vi "Przebiegi_edycja_math.vi"(8 "error in (no error)":errorcluster, 11 "Wektor przebiegow in":waveform(dbl)[](array[waveform])) -> (0 "error out":errorcluster, 3 "Wektor przebiegow out":waveform(dbl)[](array[waveform]))   [LabVIEW 2013]
doc: "Realizuje funkcję\nf(x) = a * sygnał + b\nna wybranym przebiegu"
panel:
  in  "C":dbl
  in  "Przebieg C":i32(ring) items=["Przebieg 0", "Przebieg 1", "Przebieg 2", "Przebieg 3", "Stała"]
  in  "Przebieg B":i32(ring) items=["Przebieg 0", "Przebieg 1", "Przebieg 2", "Przebieg 3", "Stała"]
  out "Funkcja":string
  in  "B":dbl=1.0
  in  "A":dbl=1.0
  in  "OK Button":bool
  in  "Cancel Button":bool
  in  "Przebieg A":i32(ring) items=["Przebieg 0", "Przebieg 1", "Przebieg 2", "Przebieg 3", "Stała"]
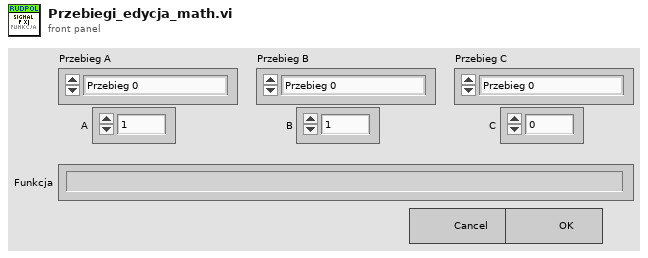
[diagram p1: front panel]
types:
  T1 = cluster{"Przebieg A":i32, "Przebieg B":i32, "Przebieg C":i32, "A":dbl, "B":dbl, "C":dbl}
  T2 = typedef "LVStringsAndValuesArrayTypeDef_I32.ctl" = cluster{"String":string, "Value":i32}[]
  T3 = cluster{"StringsAndValues[]":T2, "StringsAndValues[]":T2, "StringsAndValues[]":T2}
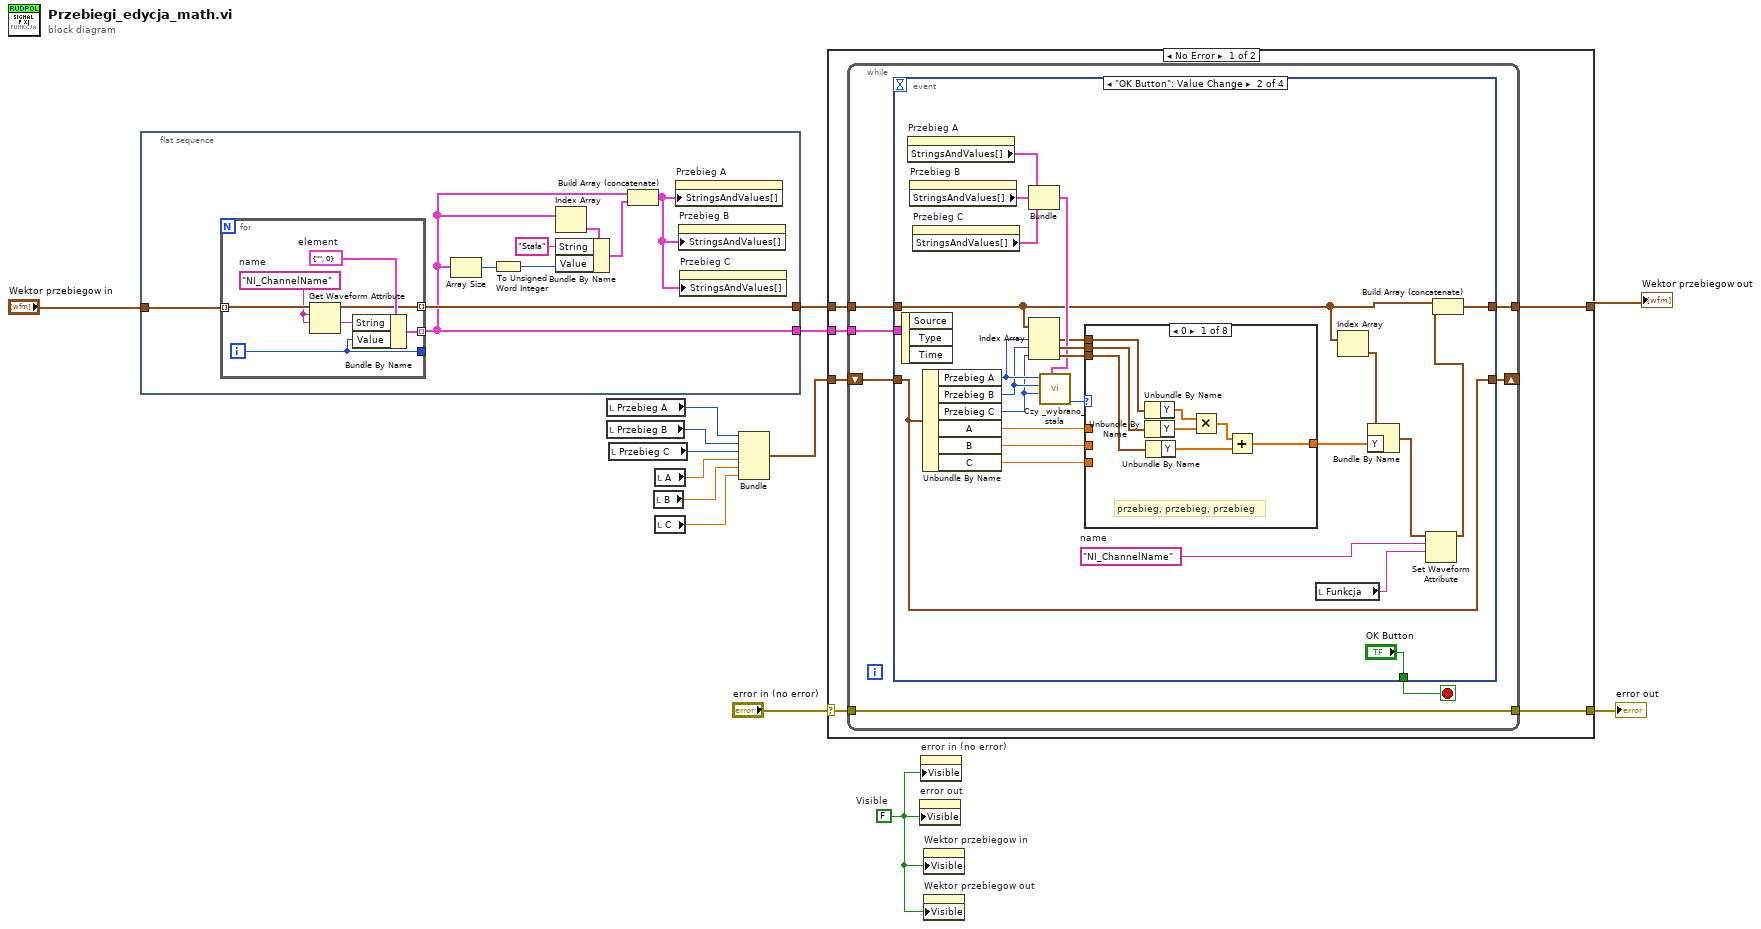
[diagram p0: block diagram]
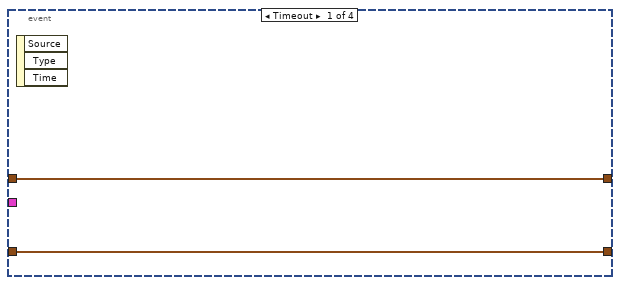
[diagram p2: hidden frame]
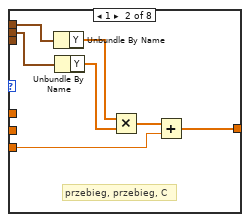
[diagram p3: hidden frame]
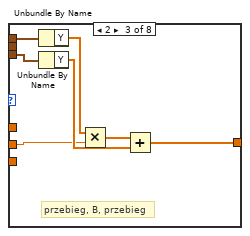
[diagram p4: hidden frame]
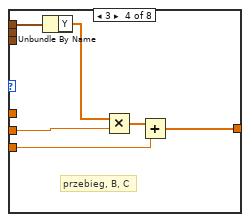
[diagram p5: hidden frame]
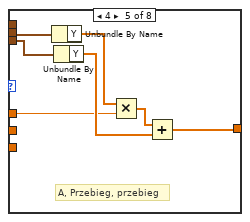
[diagram p6: hidden frame]
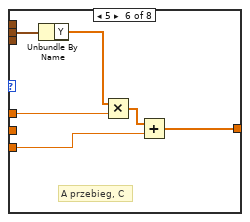
[diagram p7: hidden frame]
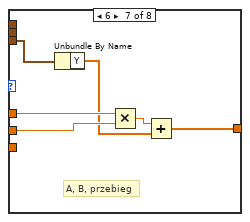
[diagram p8: hidden frame]
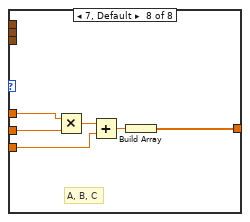
[diagram p9: hidden frame]
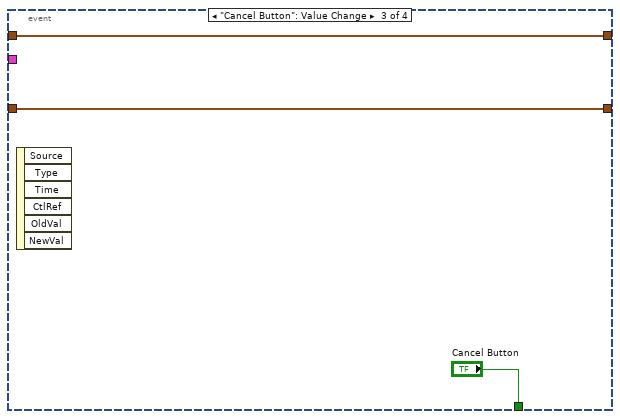
[diagram p10: hidden frame]
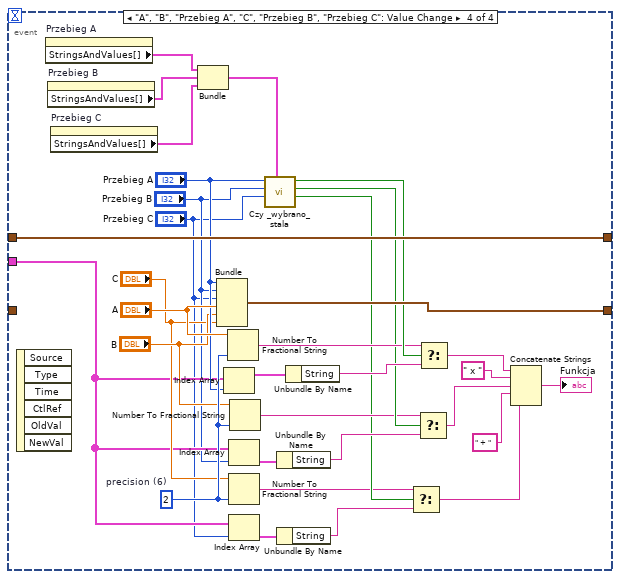
[diagram p11: hidden frame]
diagram:
  w8 = FALSE  # Visible
  n1 = flat-sequence {
    tunnel: "Wektor przebiegow in" -> [w23]
    tunnel: [w18] -> w11
    tunnel: [w22] -> w10
    frame #0 {
      n2 = for {
        tunnel: w23 -> [w30] mode=indexing
        tunnel: [w26] -> _
        tunnel: [w25] -> w18 mode=indexing
        tunnel: [w24] -> w22 mode=indexing
        i -> [w26]
        w28 = cluster{"String":string, "Value":u16} {"String"="", "Value"=0}  # element
        w29 = "NI_ChannelName"  # name
        n3 = Get Waveform Attribute(5:w29, 6:w29, 7:w30) -> (1:w27:string, 3:w24:waveform(dbl))  [unwired: 1 in, 2 out]
        n4 = Bundle By Name(cluster=w28, "String"=w27, "Value"=w26) -> (w25:cluster{"String":string, "Value":u16})
      }
      n5 = Array Size(array=w18) -> (size(s)=w17:i32)
      n6 = To Unsigned Word Integer(number=w17) -> (unsigned 16bit integer=w16:u16)
      n7 = Index Array(array=w18) -> (element=w21:cluster{"String":string, "Value":u16})  [unwired: 1 in]
      n8 = Bundle By Name(cluster=w21, "String"="Stała", "Value"=w16) -> (w20:cluster{"String":string, "Value":u16})
      n9 = Build Array (concatenate)(w18, w20) -> (w15:cluster{"String":string, "Value":u16}[])
      n10 = property on="Przebieg A" class="Ring (strict)"("StringsAndValues[]"=w15) -> ()  [unwired: 2 in, 2 out]
      n11 = property on="Przebieg B" class="Ring (strict)"("StringsAndValues[]"=w15) -> ()  [unwired: 2 in, 2 out]
      n12 = property on="Przebieg C" class="Ring (strict)"("StringsAndValues[]"=w15) -> ()  [unwired: 2 in, 2 out]
    }
  }
  n13 = local read "Przebieg A"() -> (w7:i32)
  n14 = local read "Przebieg B"() -> (w2:i32)
  n15 = local read "Przebieg C"() -> (w1:i32)
  n16 = local read "B"() -> (w4:dbl)
  n17 = local read "A"() -> (w5:dbl)
  n18 = local read "C"() -> (w3:dbl)
  n19 = Bundle("Przebieg A"=w7, "Przebieg B"=w2, "Przebieg C"=w1, "A"=w5, "B"=w4, "C"=w3) -> (w6:T1)  [unwired: 1 in]
  n20 = case shown="No Error" "error in (no error)" {
    selector: "error in (no error)" -> [w34 w159]
    tunnel: [w33 w159] -> w13
    tunnel: w11 -> [w32 _]
    tunnel: w10 -> [w36 w158]
    tunnel: [w35 w158] -> w9
    tunnel: w6 -> [w31 _]
    frame No Error {
      n21 = while {
        tunnel: w36 -> [w43]
        tunnel: [w42] -> w35
        tunnel: w34 -> [w40]
        tunnel: [w40] -> w33
        shift-right: [w39] -> _
        shift-left: w31 -> [w38]
        tunnel: w32 -> [w37]
        stop <- w41 stop-if-true
        n22 = event shown="[1] \"OK Button\": Value Change" {
          selector: _ -> [_ _ _ _]
          dyn-events: _ -> [_ _ _ _]
          timeout: _ -> [_ _ _ _]
          tunnel: w43 -> [w44 w47 w125 w152]
          tunnel: [w44 w68 w125 w152] -> w42
          tunnel: [_ "OK Button" "Cancel Button" _] -> w41
          tunnel: [w45 w63 w123 w157] -> w39
          tunnel: w38 -> [w45 w63 w123 _]
          tunnel: w37 -> [_ _ _ w133]
          event Timeout {
            n23 = event-data() -> ()  [unwired: 1 in, 3 out]
          }
          event "OK Button": Value Change {
            w65 = "NI_ChannelName"  # name
            n24 = event-data() -> ()  [unwired: 1 in, 3 out]
            n25 = property on="Przebieg A" class="Ring (strict)"() -> ("StringsAndValues[]"=w52:T2)  [unwired: 2 in, 2 out]
            n26 = property on="Przebieg B" class="Ring (strict)"() -> ("StringsAndValues[]"=w51:T2)  [unwired: 2 in, 2 out]
            n27 = property on="Przebieg C" class="Ring (strict)"() -> ("StringsAndValues[]"=w50:T2)  [unwired: 2 in, 2 out]
            n28 = Unbundle By Name(w63) -> ("Przebieg A"=w62:i32, "Przebieg B"=w61:i32, "Przebieg C"=w60:i32, "A"=w59:dbl, "B"=w55:dbl, "C"=w54:dbl)
            n29 = Bundle("StringsAndValues[]"=w52, "StringsAndValues[]"=w51, "StringsAndValues[]"=w50) -> (w49:T3)  [unwired: 1 in]
            n30 = Index Array(array=w47, index #1=w62, index #2=w61, index #3=w60) -> (element #1=w48:waveform(dbl), element #2=w57:waveform(dbl), element #3=w56:waveform(dbl))
            n31 = call "Czy _wybrano_stala.vi"("output cluster"=w49, "Przebieg C"=w60, "Przebieg B"=w61, "Przebieg A"=w62) -> ("akcja"=w58:u8)  [unwired: 4 in, 3 out]
            n32 = case shown="0" w58 {
              tunnel: w59 -> [_ _ _ _ w98 w107 w114 w122]
              tunnel: w48 -> [w77 w81 w88 w97 _ _ _ _]
              tunnel: w57 -> [w76 w80 _ _ w104 w110 _ _]
              tunnel: w56 -> [w75 _ w87 _ w103 _ w115 _]
              tunnel: w55 -> [_ _ w85 w95 _ _ w113 w121]
              tunnel: w54 -> [_ w83 _ w93 _ w108 _ w119]
              tunnel: [w70 w84 w89 w92 w101 w105 w111 w117] -> w53
              frame 0 {
                # "przebieg, przebieg, przebieg"
                n33 = Unbundle By Name(w77) -> ("Y"=w74:dbl[])
                n34 = Unbundle By Name(w76) -> ("Y"=w73:dbl[])
                n35 = Unbundle By Name(w75) -> ("Y"=w71:dbl[])
                n36 = Multiply(x=w74, y=w73) -> (x*y=w72:dbl[])
                n37 = Add(x=w72, y=w71) -> (x+y=w70:dbl[])
              }
              frame 1 {
                # "przebieg, przebieg, C"
                n38 = Unbundle By Name(w81) -> ("Y"=w78:dbl[])
                n39 = Unbundle By Name(w80) -> ("Y"=w79:dbl[])
                n40 = Multiply(x=w78, y=w79) -> (x*y=w82:dbl[])
                n41 = Add(x=w82, y=w83) -> (x+y=w84:dbl[])
              }
              frame 2 {
                # "przebieg, B, przebieg"
                n42 = Unbundle By Name(w88) -> ("Y"=w91:dbl[])
                n43 = Unbundle By Name(w87) -> ("Y"=w86:dbl[])
                n44 = Multiply(x=w91, y=w85) -> (x*y=w90:dbl[])
                n45 = Add(x=w90, y=w86) -> (x+y=w89:dbl[])
              }
              frame 3 {
                # "przebieg, B, C"
                n46 = Unbundle By Name(w97) -> ("Y"=w96:dbl[])
                n47 = Multiply(x=w96, y=w95) -> (x*y=w94:dbl[])
                n48 = Add(x=w94, y=w93) -> (x+y=w92:dbl[])
              }
              frame 4 {
                # "A, Przebieg, przebieg"
                n49 = Unbundle By Name(w104) -> ("Y"=w99:dbl[])
                n50 = Unbundle By Name(w103) -> ("Y"=w100:dbl[])
                n51 = Multiply(x=w99, y=w98) -> (x*y=w102:dbl[])
                n52 = Add(x=w102, y=w100) -> (x+y=w101:dbl[])
              }
              frame 5 {
                # "A przebieg, C"
                n53 = Unbundle By Name(w110) -> ("Y"=w106:dbl[])
                n54 = Multiply(x=w106, y=w107) -> (x*y=w109:dbl[])
                n55 = Add(x=w109, y=w108) -> (x+y=w105:dbl[])
              }
              frame 6 {
                # "A, B, przebieg"
                n56 = Unbundle By Name(w115) -> ("Y"=w112:dbl[])
                n57 = Multiply(x=w114, y=w113) -> (x*y=w116:dbl)
                n58 = Add(x=w116, y=w112) -> (x+y=w111:dbl[])
              }
              frame 7, Default {
                # "A, B, C"
                n59 = Multiply(x=w122, y=w121) -> (x*y=w120:dbl)
                n60 = Add(x=w120, y=w119) -> (x+y=w118:dbl)
                n61 = Build Array(w118) -> (w117:dbl[])
              }
            }
            n62 = local read "Funkcja"() -> (w66:string)
            n63 = Index Array(array=w47) -> (element=w46:waveform(dbl))  [unwired: 1 in]
            n64 = Bundle By Name(cluster=w46, "Y"=w53) -> (w67:waveform(dbl))
            n65 = Set Waveform Attribute(5:w66, 6:w65, 7:w67) -> (3:w64:waveform(dbl))  [unwired: 1 in, 2 out]
            n66 = Build Array (concatenate)(w47, w64) -> (w68:waveform(dbl)[])
          }
          event "Cancel Button": Value Change {
            n67 = event-data() -> ()  [unwired: 1 in, 6 out]
          }
          event "A", "B", "Przebieg A", "C", "Przebieg B", "Przebieg C": Value Change {
            w151 = i16 2  # precision (6)
            n68 = event-data() -> ()  [unwired: 1 in, 6 out]
            n69 = property on="Przebieg A" class="Ring (strict)"() -> ("StringsAndValues[]"=w149:T2)  [unwired: 2 in, 2 out]
            n70 = property on="Przebieg B" class="Ring (strict)"() -> ("StringsAndValues[]"=w148:T2)  [unwired: 2 in, 2 out]
            n71 = property on="Przebieg C" class="Ring (strict)"() -> ("StringsAndValues[]"=w147:T2)  [unwired: 2 in, 2 out]
            n72 = Bundle("StringsAndValues[]"=w149, "StringsAndValues[]"=w148, "StringsAndValues[]"=w147) -> (w146:T3)  [unwired: 1 in]
            n73 = Bundle("Przebieg A"="Przebieg A", "Przebieg B"="Przebieg B", "Przebieg C"="Przebieg C", "A"="A", "B"="B", "C"="C") -> (w157:T1)  [unwired: 1 in]
            n74 = Index Array(array=w133, index="Przebieg A") -> (element=w154:cluster{"String":string, "Value":u16})
            n75 = Number To Fractional String(number="A", precision (6)=w151) -> (F-format string=w143:string)  [unwired: 2 in]
            n76 = Index Array(array=w133, index="Przebieg B") -> (element=w139:cluster{"String":string, "Value":u16})
            n77 = Number To Fractional String(number="C", precision (6)=w151) -> (F-format string=w127:string)  [unwired: 2 in]
            n78 = Index Array(array=w133, index="Przebieg C") -> (element=w130:cluster{"String":string, "Value":u16})
            n79 = Number To Fractional String(number="B", precision (6)=w151) -> (F-format string=w137:string)  [unwired: 2 in]
            n80 = call "Czy _wybrano_stala.vi"("output cluster"=w146, "Przebieg C"="Przebieg C", "Przebieg B"="Przebieg B", "Przebieg A"="Przebieg A") -> ("Stala C?"=w129:bool, "Stala B?"=w138:bool, "Stala A?"=w144:bool)  [unwired: 4 in, 1 out]
            n81 = Unbundle By Name(w139) -> ("String"=w136:string)
            n82 = Unbundle By Name(w130) -> ("String"=w128:string)
            n83 = Unbundle By Name(w154) -> ("String"=w142:string)
            n84 = Select(t=w127, s=w129, f=w128) -> (s? t:f=w126:string)
            n85 = Select(t=w137, s=w138, f=w136) -> (s? t:f=w135:string)
            n86 = Select(t=w143, s=w144, f=w142) -> (s? t:f=w141:string)
            n87 = Concatenate Strings(w141, " x " ("string"), w135, " + " ("string"), w126) -> (→"Funkcja":string)
          }
        }
      }
    }
    frame Error {
    }
  }
  "error out" <- w13
  "Wektor przebiegow out" <- w9
  n88 = property on="error out" class="Clust (strict)"("Visible"=w8) -> ()  [unwired: 2 in, 2 out]
  n89 = property on="error in (no error)" class="Clust (strict)"("Visible"=w8) -> ()  [unwired: 2 in, 2 out]
  n90 = property on="Wektor przebiegow in" class="Arr (strict)"("Visible"=w8) -> ()  [unwired: 2 in, 2 out]
  n91 = property on="Wektor przebiegow out" class="Arr (strict)"("Visible"=w8) -> ()  [unwired: 2 in, 2 out]
